vi "MouseUp Response.vi"(4 "PlatMods":T1, 6 "Mods":cluster{"Double Click":bool, "Menu Key":bool}, 8 "error in (no error)":errorcluster, 9 "Button":u16, 10 "Coords":T2, 11 "Editor Handler in":refnum<class "3DButton Handler.lvclass">) -> (0 "error out":errorcluster, 3 "Editor Handler out":refnum<class "3DButton Handler.lvclass">)   [LabVIEW 2016, in "3DButton Handler.lvclass"]
uses:
  3DButton Handler.lvclass
  C:/Program Files (x86)/National Instruments/LabVIEW 2016/vi.lib/LIEF/Image Editor Handler/Image Editor Handler.lvclass
  <vilib>/Utility/miscctls.llb/LVPoint32TypeDef.ctl
  <vilib>/LIEF/Image Editor Handler/Image Editor Handler.lvclass/Image Editor Handler.ctl
  <vilib>/LIEF/Forms/Selection/Selection.lvclass
  C:/Program Files (x86)/National Instruments/LabVIEW 2016/vi.lib/LIEF/Forms/Shape/Shape.lvclass
  Rectangle3D/Rectangle3D.lvclass
  <vilib>/LIEF/Forms/Selection/Selection.lvclass/Selection.ctl
  Rectangle3D/Rectangle3D.lvclass/Rectangle3D.ctl
  Rectangle3D/Write Clicked.vi
  <vilib>/LIEF/Forms/Selection/Read Selected Shape.vi
  <vilib>/LIEF/Image Editor Handler/Write Shapes.vi
  <vilib>/LIEF/Image Editor Handler/Read PictureRef.vi
  <vilib>/LIEF/Image Editor Handler/Read Shapes.vi
  <vilib>/LIEF/Forms/Shape/Shape.lvclass
  <vilib>/LIEF/Image Editor Handler/Image Editor Handler.lvclass
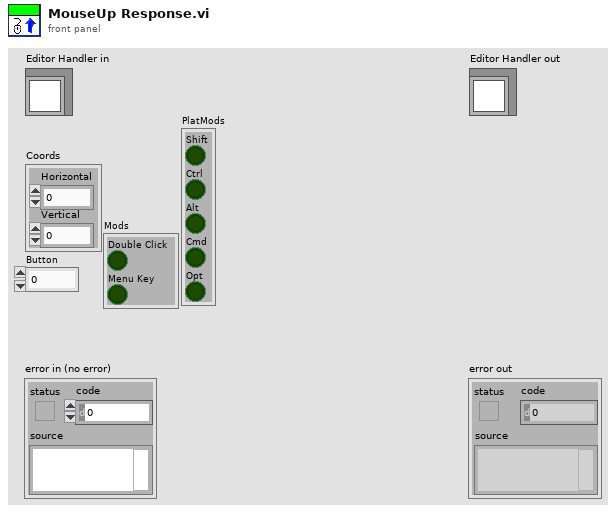
[diagram p1: front panel]
types:
  T1 = cluster{"Shift":bool, "Ctrl":bool, "Alt":bool, "Cmd":bool, "Opt":bool}
  T2 = typedef "LVPoint32TypeDef.ctl" = cluster{"Horizontal":i32, "Vertical":i32}
  T3 = typedef "LVPositionTypeDef.ctl" = cluster{"Left":i32, "Top":i32}
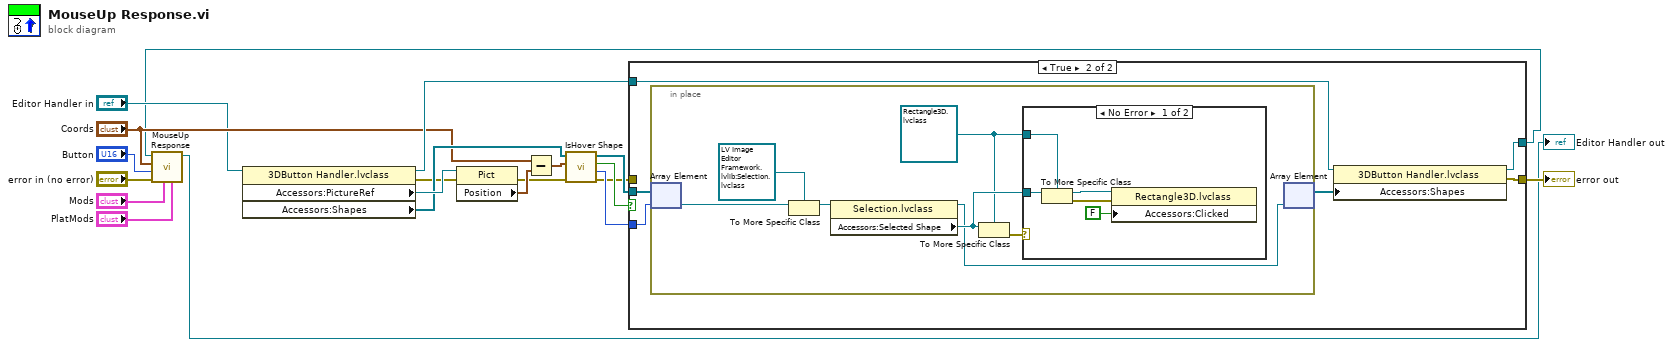
[diagram p0: block diagram]
diagram:
  n1 = property class="3DButton Handler.lvclass"(reference="Editor Handler in") -> (reference out=w12:refnum<class "3DButton Handler.lvclass">, error out=w7:errorcluster, "Accessors:PictureRef"=w14:refnum<vi>, "Accessors:Shapes"=w13:refnum<data-value>[])  [unwired: 1 in]
  n2 = property class="Pict"(reference=w14, error in=w7) -> (error out=w15:errorcluster, "Position"=w17:T3)  [unwired: 1 out]
  n3 = Subtract(x="Coords", y=w17) -> (x-y=w16:T2)
  n4 = call <vilib>:"IsHover Shape.vi"("error in (no error)"=w15, "Coords"=w16, "Shape in"=w13) -> ("error out"=w8:errorcluster, "Node ID"=w10:i32, "Found?"=w9:bool, "Shape out"=w11:refnum<data-value>[])  [unwired: 3 in, 2 out]
  n5 = case shown="True" w9 {
    tunnel: w12 -> [w22 w28]
    tunnel: w11 -> [_ w27]
    tunnel: w10 -> [_ w26]
    tunnel: [w22 w24] -> w2
    tunnel: [w21 w23] -> w4
    tunnel: w8 -> [w21 _]
    frame False {
    }
    frame True {
      n6 = in-place {
        w30 = refnum<data-value> refnum ("target class")
        n7 = in-place-array #1(w27, w26) -> (w35:refnum<data-value>)
        n8 = To More Specific Class(target class=refnum<data-value> refnum, reference=w35) -> (specific class reference=w33:refnum<data-value>)  [unwired: 1 in, 1 out]
        n9 = property class="Selection.lvclass"(reference=w33) -> (reference out=w29:refnum<data-value>, "Accessors:Selected Shape"=w31:refnum<data-value>)  [unwired: 1 in, 1 out]
        n10 = To More Specific Class(target class=w30, reference=w31) -> (error out=w32:errorcluster)  [unwired: 1 in, 1 out]
        n11 = case shown="No Error" w32 {
          tunnel: w31 -> [w39 _]
          tunnel: w30 -> [w38 _]
          frame No Error {
            n12 = To More Specific Class(target class=w38, reference=w39) -> (specific class reference=w37:refnum<data-value>, error out=w40:errorcluster)  [unwired: 1 in]
            n13 = property class="Rectangle3D.lvclass"(reference=w37, error in=w40, "Accessors:Clicked"=FALSE ("Clicked")) -> ()  [unwired: 2 out]
          }
          frame Error {
          }
        }
        n14 = in-place-array #1(w29) -> (w25:refnum<data-value>[])  [unwired: 1 out]
      }
      n15 = property class="3DButton Handler.lvclass"(reference=w28, "Accessors:Shapes"=w25) -> (reference out=w24:refnum<class "3DButton Handler.lvclass">, error out=w23:errorcluster)  [unwired: 1 in]
    }
  }
  "error out" <- w4
  n16 = call-parent "MouseUp Response.vi"("PlatMods"="PlatMods", "Mods"="Mods", "error in (no error)"="error in (no error)", "Button"="Button", "Coords"="Coords", "Editor Handler in"=w2) -> ("Editor Handler out"=→"Editor Handler out":refnum<class "3DButton Handler.lvclass">)  [unwired: 4 in, 1 out]
